vi "TaskInitialize.vi"(8 "error in (no error)":errorcluster, 11 "HGF_DSCVarManager in":refnum<class "HGF_DSCVarManager.lvclass">) -> (0 "error out":errorcluster, 3 "HGF_DSCVarManager out":refnum<class "HGF_DSCVarManager.lvclass">)   [LabVIEW 2012, in "HGF_DSC.lvlib" / "HGF_DSCVarManager.lvclass"]
doc: "Called by TaskLoop to initialize Task.\nCreates a Process for this Variable Manager and returns a warning, if defined process name already exists\n\nF.Berck@gsi.de\nGSI Darmstadt 2010"
uses:
  HGF_DSCVarManager.lvclass
  HGF_DSCVarManager.lvclass/HGF_DSCVarManager.ctl
  HGF_BaseClasses/HGF_Factory/HGF_Factory.lvclass
  <vilib>/lvdsc/NI_DSC.lvlib
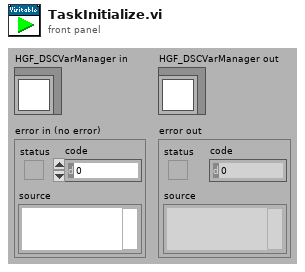
[diagram p1: front panel]
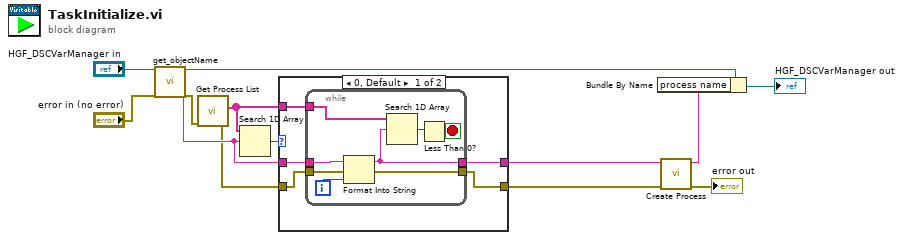
[diagram p0: block diagram]
diagram:
  n1 = call "get_objectName.vi"("HGF_Factory"="HGF_DSCVarManager in", "error in (no error)"="error in (no error)") -> ("dup HGF_Factory"=w10:refnum<class "HGF_DSCVarManager.lvclass">, "objectName"=w13:string, "error out"=w11:errorcluster)  [unwired: 15 out]
  n2 = call <vilib>:"Get Process List.vi"("error in (no error)"=w11) -> ("error out"=w3:errorcluster, "processes"=w6:string[])  [unwired: 9 out]
  n3 = Search 1D Array(1D array=w6, element=w13) -> (index of element=w12:i32)  [unwired: 1 out]
  n4 = case shown="0, Default" w12 {
    tunnel: w13 -> [w17 w28]
    tunnel: [w16 w28] -> w4
    tunnel: w6 -> [w18 _]
    tunnel: w3 -> [w15 w27]
    tunnel: [w14 w27] -> w2
    frame 0, Default {
      n5 = while {
        tunnel: w18 -> [w26]
        tunnel: w17 -> [w23]
        tunnel: [w21] -> w16
        tunnel: w15 -> [w20]
        tunnel: [w19] -> w14
        i -> [w22]
        stop <- w24 stop-if-true
        n6 = Format Into String(initial string=w23, error in=w20, w22) -> (resulting string=w21:string, error out=w19:errorcluster)  [unwired: 1 in]
        n7 = Search 1D Array(1D array=w26, element=w21) -> (index of element=w25:i32)  [unwired: 1 out]
        n8 = Less Than 0?(x=w25) -> (x < 0?=w24:bool)
      }
    }
    frame -1 {
    }
  }
  n9 = call <vilib>:"Create Process.vi"("error in (no error)"=w2, "process name"=w4) -> ("error out"=→"error out":errorcluster, "process name out"=w5:string)  [unwired: 4 in, 4 out]
  n10 = Bundle By Name(cluster=w10, "process name"=w5) -> (→"HGF_DSCVarManager out":refnum<class "HGF_DSCVarManager.lvclass">)
